vi "set-B-field.vi"(7 "upper limit":dbl=2.906, 8 "physical channels":tag="Dev1/ao0", 9 "Coil supply":enum16{"KEPCO", "BOUHNIK", "NONE"}(ring), 10 "Field (T)":dbl min=0.0 max=16.0, 11 "GPIB adr in":string) -> (3 "GPIB adr out":string)   [LabVIEW 2010]
doc: "Sets the coil filed (assuming 120A mode on power supply).\nGive B value as positive number, and set the sign via the polarity\nconnector (true = plus sign)."
uses:
  <vilib>/DAQmx/write.llb/DAQmx Write (Analog DBL 1Chan 1Samp).vi
  <vilib>/DAQmx/create/channels.llb/DAQmx Create Channel (AO-Voltage-Basic).vi
  <vilib>/daqmx/miscellaneous.llb/DAQmx Fill In Error Info.vi
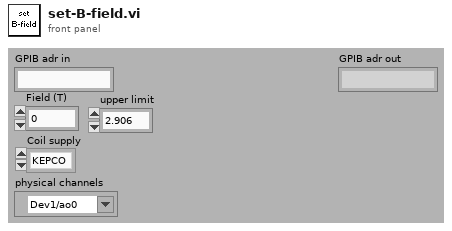
[diagram p1: front panel]
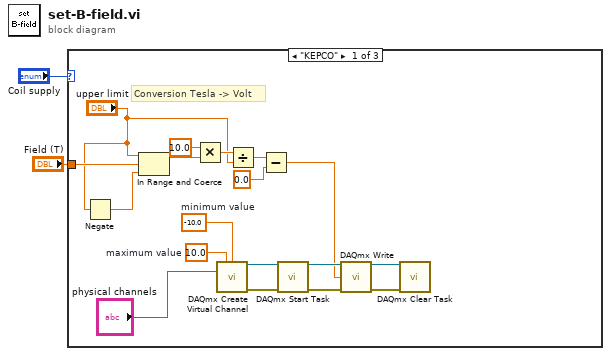
[diagram p0: block diagram]
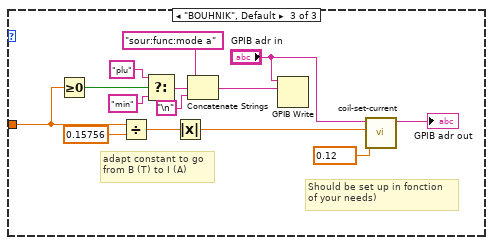
[diagram p3: hidden frame]
diagram:
  n1 = case shown="\"KEPCO\"" "Coil supply" {
    tunnel: "Field (T)" -> [w11 _ w22]
    frame "KEPCO" {
      w12 = 10.0  # maximum value
      w13 = -10.0  # minimum value
      # "Conversion Tesla -> Volt"
      n2 = Negate(x="upper limit") -> (-x=w4:dbl)
      n3 = In Range and Coerce(upper limit="upper limit", x=w11, lower limit=w4) -> (coerced(x)=w10:dbl)  [unwired: 1 out]
      n4 = Multiply(x=10.0, y=w10) -> (x*y=w8:dbl)
      n5 = call-poly <vilib>:"DAQmx Create Virtual Channel.vi"("maximum value"=w12, "minimum value"=w13, "physical channels"="physical channels") -> ("task out"=w19:refnum<k21>, "error out"=w18:errorcluster)  [unwired: 6 in, 5 out]
      n6 = Divide(x=w8, y="upper limit") -> (x/y=w7:dbl)
      n7 = Subtract(x=w7, y=0.0) -> (x-y=w6:dbl)
      n8 = call <vilib>:"DAQmx Start Task.vi"("task/channels in"=w19, "error in"=w18) -> ("task out"=w17:refnum<k21>, "error out"=w16:errorcluster)  [unwired: 12 out]
      n9 = call-poly <vilib>:"DAQmx Write.vi"("task/channels in"=w17, "data"=w6, "error in"=w16) -> ("task out"=w15:refnum<k21>, "error out"=w14:errorcluster)  [unwired: 1 in, 10 out]
      n10 = call <vilib>:"DAQmx Clear Task.vi"("task in"=w15, "error in"=w14) -> ()  [unwired: 14 out]
    }
    frame "NONE" {
    }
    frame "BOUHNIK", Default {
      w30 = 0.12 items=["12A"=0.012, "120A"=0.12] ("mode")
      # "adapt constant to go\nfrom B (T) to I (A)"
      # "Should be set up in fonction\nof your needs)"
      n11 = Greater Or Equal To 0?(x=w22) -> (x >= 0?=w21:bool)
      n12 = Divide(x=w22, y=0.15756) -> (x/y=w32:dbl)
      n13 = Select(t="plu" ("GPIB adr in"), s=w21, f="min" ("GPIB adr in")) -> (s? t:f=w26:string)
      n14 = Absolute Value(x=w32) -> (abs(x)=w29:dbl)
      n15 = Concatenate Strings("sour:func:mode a" ("string"), w26, "\n") -> (w23:string)
      n16 = GPIB Write(0:"GPIB adr in", 1:w23) -> ()  [unwired: 1 in, 4 out]
      n17 = call "coil-set-current.vi"("mode"=w30, "Current (A)"=w29, "GPIB adr in"="GPIB adr in") -> ("GPIB adr out"=→"GPIB adr out":string)  [unwired: 8 out]
    }
  }
